vi "DriverStationGetData.vi"   [LabVIEW 2018]
uses:
  <vilib>/Rock Robotics/Network Tables/NT Read Boolean.vi
  dsdata.vi
  <vilib>/Rock Robotics/Network Tables/NT Read String.vi
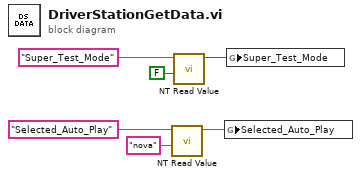
[diagram p0: block diagram]
diagram:
  n1 = call-poly <vilib>:"NT Read Value.vi"("Default Value"="nova", "Name"="Selected_Auto_Play" ("refnum name")) -> ("String"=w1:string)  [unwired: 8 in, 1 out]
  n2 = call-poly <vilib>:"NT Read Value.vi"("Default Value"=FALSE, "Name"="Super_Test_Mode" ("refnum name")) -> ("Boolean"=w4:bool)  [unwired: 8 in, 1 out]
  n3 = global write "dsdata.vi" "Selected_Auto_Play"(w1) -> ()
  n4 = global write "dsdata.vi" "Super_Test_Mode"(w4) -> ()
